vi "Create BooleanArrayMsg.vi"(8 "error in (no error)":errorcluster, 10 "Message Data":bool[](array[boolean]), 11 "Message Name":string) -> (0 "error out":errorcluster, 3 "BooleanArrayMsg out":refnum<class "BooleanArrayMsg.lvclass">)   [LabVIEW 2009, in "LapDog.Messaging.v2.NativeArrays.lvlib" / "BooleanArrayMsg.lvclass"]
doc: "Returns a BooleanArrayMsg object with the given name.\n\nThis method executes regardless of the error in state."
uses:
  BooleanArrayMsg.lvclass
  BooleanArrayMsg.lvclass/BooleanArrayMsg.ctl
  Messaging.v2/MessageObject/Message.lvclass
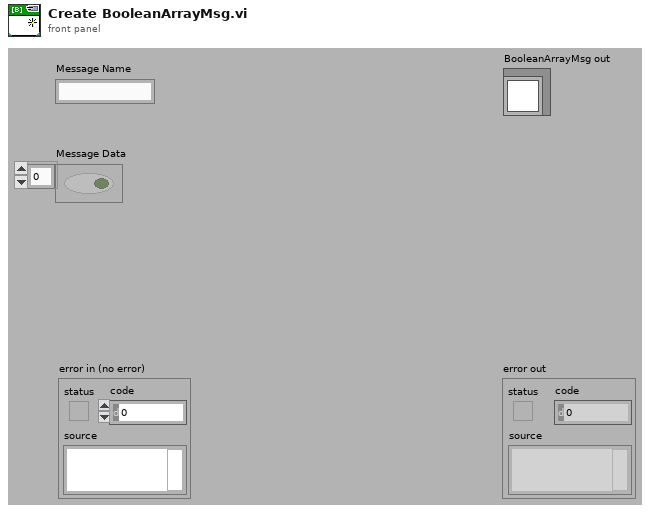
[diagram p1: front panel]
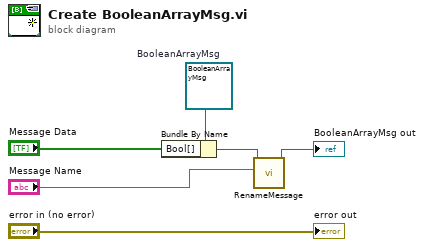
[diagram p0: block diagram]
diagram:
  w5 = refnum<class "BooleanArrayMsg.lvclass"> refnum  # BooleanArrayMsg
  n1 = Bundle By Name(cluster=w5, "Bool[]"="Message Data") -> (w3:refnum<class "BooleanArrayMsg.lvclass">)
  n2 = call "RenameMessage.vi"("Message Name"="Message Name", "Message in"=w3) -> ("Message out"=→"BooleanArrayMsg out":refnum<class "BooleanArrayMsg.lvclass">)  [unwired: 8 in, 1 out]
  "error out" <- "error in (no error)"
